vi "Initialize PSU.vi"(8 "error in":errorcluster, 9 "Field Constant":dbl, 11 "PSU VISA name":refnum<visa-resource-name>) -> (0 "error out":errorcluster, 1 "Initial message":string, 2 "initial PSU Status":T1 {"Trip Current" format="%.3f"; "Trip Field" format="%.4f"; "Voltage" format="%.2f"; "Field Constant" format="%.6f"; "MID Setpoint (T)" format="%.4f"; "MID Setpoint (A)" format="%.3f"; "MAX Setpoint (T)" format="%.4f"; "MAX Setpoint (A)" format="%.3f"; "Heater Voltage" format="%.2f"; "V Limit (V)" format="%.2f"; "Ramp Rate (A/s)" format="%.3f"; "Output (A)" format="%.3f"; "Output (T)" format="%.4f"; "Persistent Current" format="%.3f"; "Persistent Field" format="%.4f"})   [LabVIEW 2022 SP3, in "Magnet module.lvlib"]
doc: "Initialize comunication with PSU and reads out whole status."
uses:
  Magnet module.lvlib
  <instrlib>/SMS 120/Public/PSU Status.ctl
  <vilib>/Utility/error.llb/Error Cluster From Error Code.vi
  <vilib>/ErrorRing/Error Ring.xnode
  <instrlib>/SMS 120/Cryogenic Ltd SMSXXX.lvlib
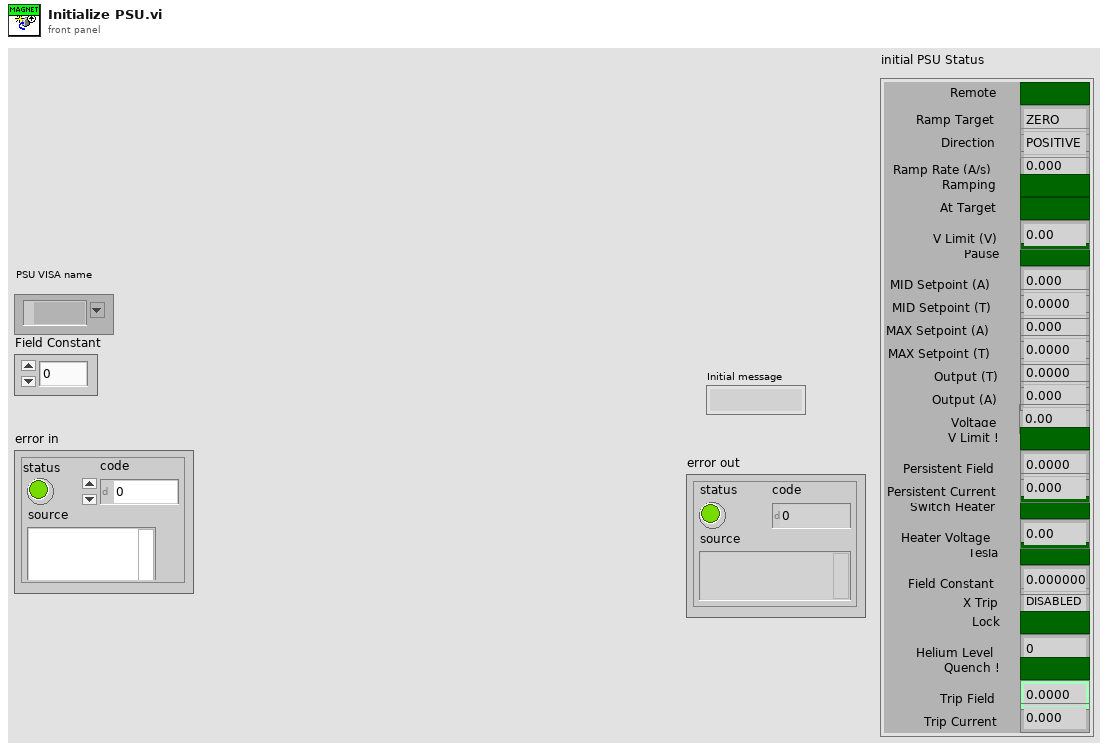
[diagram p1: front panel]
types:
  T1 = typedef "Cryogenic Ltd SMSXXX.lvlib/PSU Status.ctl" = cluster{"Ramp Target":enum16{"ZERO", "MID", "MAX"}, "Pause":bool, "Switch Heater":bool, "Persistent Field":dbl, "Persistent Current":dbl, "Tesla":bool, "Output (T)":dbl, "Output (A)":dbl, "X Trip":enum16{"DISABLED", "ENABLED", "ACTIVE"}, "Ramp Rate (A/s)":dbl, "V Limit (V)":dbl, "Heater Voltage":dbl, "MAX Setpoint (A)":dbl, "MAX Setpoint (T)":dbl, "MID Setpoint (A)":dbl, "MID Setpoint (T)":dbl, "Lock":bool, "Field Constant":dbl, "Remote":bool, "Direction":enum16{"POSITIVE", "NEGATIVE", "OPEN", "UNIPOLAR"}, "Helium Level":u16, "Quench !":bool, "Voltage":dbl, "V Limit !":bool, "Ramping":bool, "At Target":bool, "Trip Field":dbl, "Trip Current":dbl}
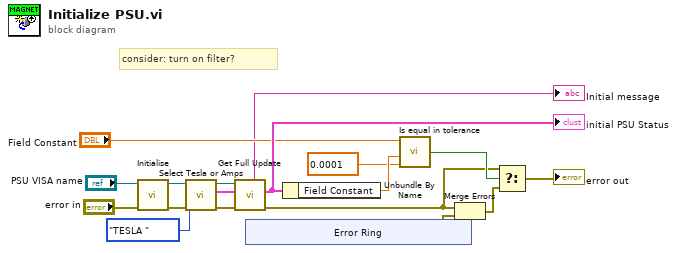
[diagram p0: block diagram]
diagram:
  # "consider: turn on filter?"
  n1 = call <instrlib>:"Initialise.vi"("error in"="error in", "SMS VISA resource name IN"="PSU VISA name") -> ("error out"=w18:errorcluster, "VISA Resource Name Out"=w3:refnum<visa-resource-name>)  [unwired: 8 in]
  n2 = call <instrlib>:"Select Tesla or Amps.vi"("Error in (no error)"=w18, "Tesla/Amps"=enum16{"AMPS", "TESLA "}."TESLA ", "VISA Resource Name In"=w3) -> ("Error out"=w5:errorcluster, "PSU Status Out"=w2:T1, "VISA Resource Name Out"=w4:refnum<visa-resource-name>)  [unwired: 5 in, 1 out]
  n3 = call <instrlib>:"Get Full Update.vi"("Error in (no error)"=w5, "PSU Status In"=w2, "VISA Resource Name In"=w4) -> ("Error out"=w7:errorcluster, "PSU Status Out"=w15:T1, "Answer"=→"Initial message":string)  [unwired: 5 in, 1 out]
  "initial PSU Status" <- w15
  n4 = xnode "Error Ring"() -> ("error out"=w10:errorcluster)
  n5 = Unbundle By Name(w15) -> ("Field Constant"=w13:dbl)
  n6 = call "Is equal in tolerance.vi"("Absolut tolerance"=0.0001, "Reference value"=w13, "Input value"="Field Constant") -> ("Is in range"=w9:bool)  [unwired: 1 in]
  n7 = Merge Errors(w7, w10) -> (w8:errorcluster)
  n8 = Select(t=w7, s=w9, f=w8) -> (s? t:f=→"error out":errorcluster)
